vi "Pre-Build Action - VxWorks.vi"(6 "Top Level/Always Included VIs":path[](array[path]), 7 "Main Destination Path":path, 9 "Target Name":string, 10 "Build Specification Name":string, 11 "Project Path":path) -> (0 "error out":errorcluster)   [LabVIEW 2011]
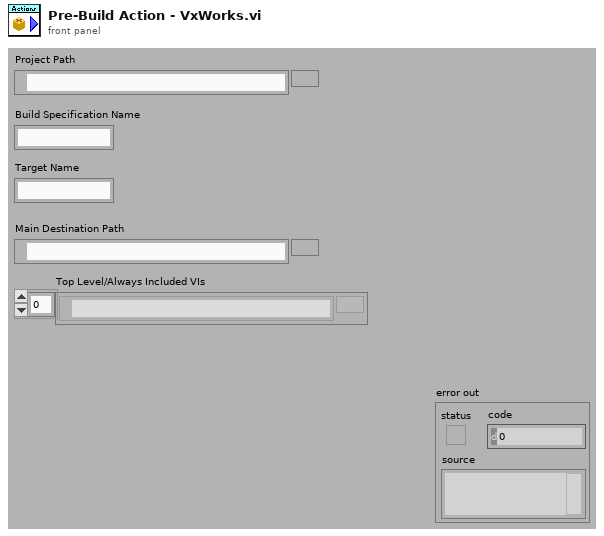
[diagram p1: front panel]
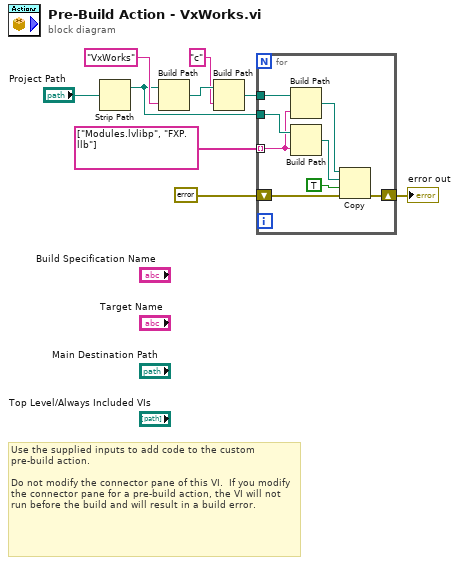
[diagram p0: block diagram]
diagram:
  # "Use the supplied inputs to add code to the custom pre-build action.\n\nDo not modify the connector pane of this VI.  If you modify the connector pane for a pre-build action, the VI will not run before the build and will result in a build error."
  n1 = Strip Path(path="Project Path") -> (stripped path=w4:path)  [unwired: 1 out]
  n2 = Build Path(base path=w4, name or relative path="VxWorks") -> (appended path=w3:path)
  n3 = Build Path(base path=w3, name or relative path="c") -> (appended path=w2:path)
  n4 = for {
    tunnel: w4 -> [w17]
    tunnel: string[] ["Modules.lvlibp", "FXP.llb"] -> [w15] mode=indexing
    tunnel: w2 -> [w16]
    shift-right: [w10] -> w6
    shift-left: errorcluster {"status"=FALSE, "code"=0, "source"=""} ("error out") -> [w11]
    n5 = Build Path(base path=w16, name or relative path=w15) -> (appended path=w14:path)
    n6 = Build Path(base path=w17, name or relative path=w15) -> (appended path=w13:path)
    n7 = Copy(8:w11, 9:TRUE ("overwrite (F)"), 10:w13, 11:w14) -> (0:w10:errorcluster)  [unwired: 1 in, 2 out]
  }
  "error out" <- w6
